vi "OAT Compensate Even Angle Signal.vi"   [LabVIEW 2017, in "SoundVib_RefDataProcess.lvlib"]
doc: "Compensates an even-angle signal. You can use the <B>compensated even-angle signal</B> output to display unfiltered orbit and timebase plots with the runout pattern removed. Wire data to the <B>even-angle signal</B> input to determine the polymorphic instance to use or manually select the instance."
uses:
  <vilib>/addons/Sound and Vibration/Order Analysis/Referece Data Processing/SoundVib_RefDataProcess.lvlib
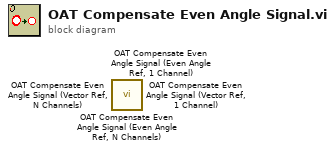
[diagram p0: block diagram]
diagram:
  n1 = call <vilib>:"OAT Compensate Even Angle Signal (Even Angle Ref, N Channels).vi"() -> ()  [unwired: 12 in, 4 out]
  n2 = call <vilib>:"OAT Compensate Even Angle Signal (Even Angle Ref, 1 Channel).vi"() -> ()  [unwired: 12 in, 4 out]
  n3 = call <vilib>:"OAT Compensate Even Angle Signal (Vector Ref, N Channels).vi"() -> ()  [unwired: 12 in, 4 out]
  n4 = call <vilib>:"OAT Compensate Even Angle Signal (Vector Ref, 1 Channel).vi"() -> ()  [unwired: 12 in, 4 out]
